vi "Exercises_6-2.vi"(1 "Power":bool) -> ()   [LabVIEW 2014]
doc: "This VI simulates measuring a temperature using the temperature sensor on the DAQ Signal Accessory.\n\nIf you have a DAQ board or a DAQ Signal Accessory, then use the Thermometer VI instead."
uses:
  Control 1.ctl
panel:
  out "Temperature History":T1
  # "ON\n\nOFF"
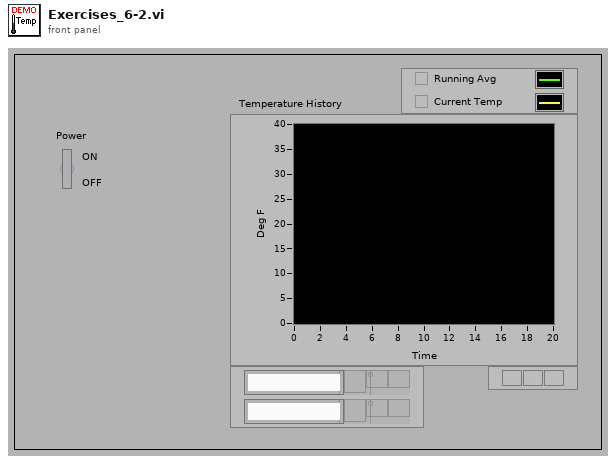
[diagram p1: front panel]
types:
  T1 = typedef "Control 1.ctl" = cluster{dbl, dbl}
  T2 = enum16{"open", "replace", "create", "open or create", "replace or create", "replace or create with confirmation"}
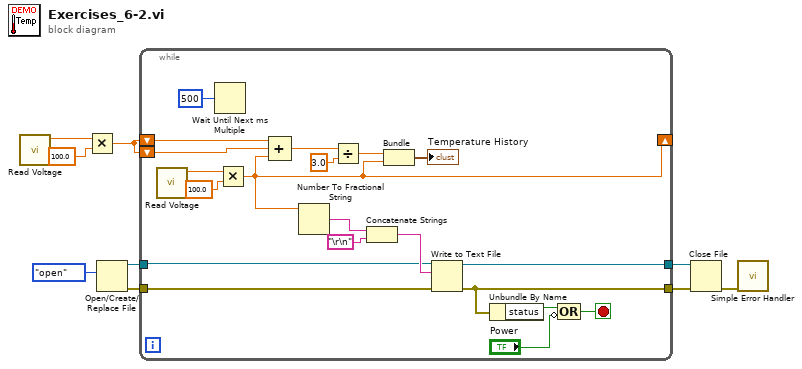
[diagram p0: block diagram]
diagram:
  n1 = call "Read Voltage.vi"() -> ("voltaje"=w1:dbl)  [unwired: 6 in, 1 out]
  n2 = Multiply(x=w1, y=100.0 ("x")) -> (x*y=w9:dbl)
  n3 = Open/Create/Replace File(operation (0:open)=T2."open") -> (refnum out=w5:refnum<file>, error out=w7:errorcluster)  [unwired: 5 in, 1 out]
  n4 = while {
    shift-right: [w11] -> _
    shift-left: w9 -> [w27]
    shift-left: w9 -> [w26]
    tunnel: w7 -> [w15]
    tunnel: [w14] -> w6
    tunnel: w5 -> [w20]
    tunnel: [w19] -> w4
    stop <- w16 stop-if-true
    n5 = call "Read Voltage.vi"() -> ("voltaje"=w13:dbl)  [unwired: 6 in, 1 out]
    n6 = Wait Until Next ms Multiple(millisecond multiple=500) -> ()  [unwired: 1 out]
    n7 = Multiply(x=w13, y=100.0 ("x")) -> (x*y=w11:dbl)
    n8 = Compound Arithmetic op=ADD(w27, w26, w11) -> (w10:dbl)
    n9 = Number To Fractional String(number=w11) -> (F-format string=w23:string)  [unwired: 3 in]
    n10 = Divide(x=w10, y=3.0) -> (x/y=w25:dbl)
    n11 = Concatenate Strings(w23, "\r\n") -> (w21:string)
    n12 = Bundle(w25, w11) -> (→"Temperature History":cluster{dbl, dbl})  [unwired: 1 in]
    n13 = Write to Text File(file (use dialog)=w20, text=w21, error in=w15) -> (refnum out=w19:refnum<file>, error out=w14:errorcluster)  [unwired: 1 in, 1 out]
    n14 = Unbundle By Name(w14) -> ("status"=w18:bool)
    n15 = Compound Arithmetic op=OR(w18, invert "Power") -> (w16:bool)
  }
  n16 = Close File(refnum=w4, error in=w6) -> (error out=w3:errorcluster)  [unwired: 1 out]
  n17 = call <vilib>:"Simple Error Handler.vi"("error in (no error)"=w3) -> ()  [unwired: 4 in, 5 out]
